vi "To Scaled Value.vi"(8 "error in":errorcluster, 10 "Response":string) -> (0 "error out":errorcluster, 1 "Unit":T1, 2 "Scaled Value":dbl format="%#.6f")   [LabVIEW 2018, in "Mercury iXX.lvlib"]
doc: "This VI converts the raw string value provided by the instrument into a scaled numeric (i.e. without prefix) and a unit string."
uses:
  Mercury iXX.lvlib
  Unit String.ctl
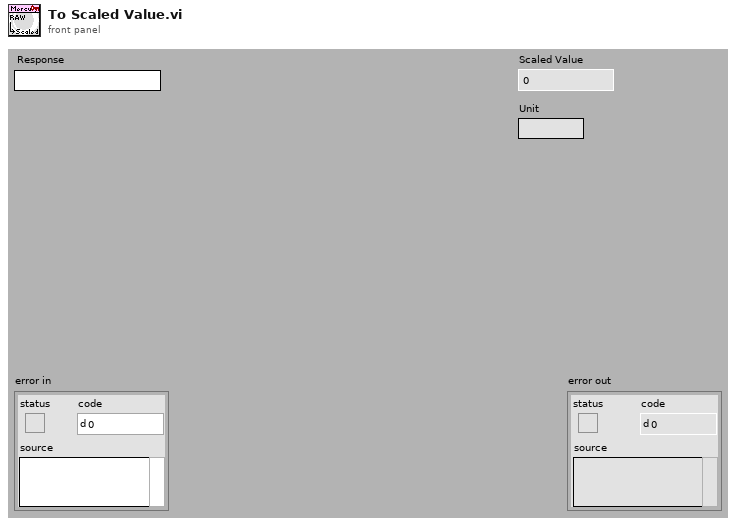
[diagram p1: front panel]
types:
  T1 = typedef "Mercury iXX.lvlib/Unit String.ctl" = string
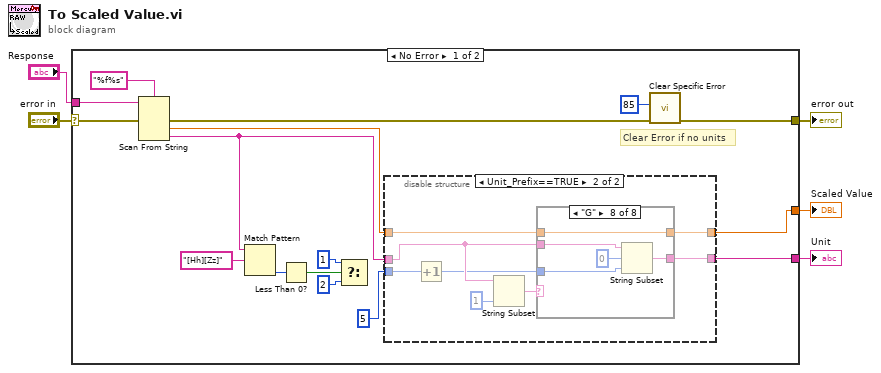
[diagram p0: block diagram]
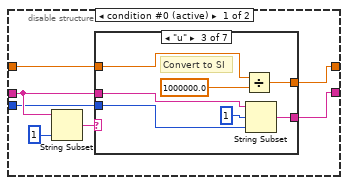
[diagram p2: hidden frame]
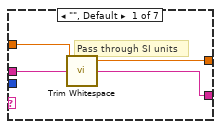
[diagram p3: hidden frame]
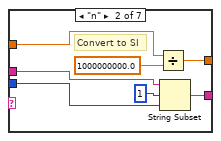
[diagram p4: hidden frame]
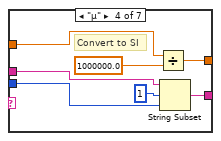
[diagram p5: hidden frame]
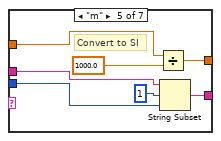
[diagram p6: hidden frame]
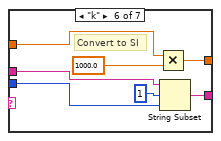
[diagram p7: hidden frame]
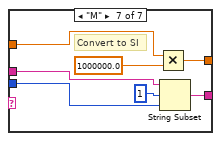
[diagram p8: hidden frame]
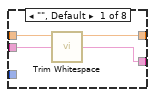
[diagram p9: hidden frame]
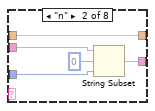
[diagram p10: hidden frame]
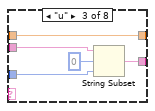
[diagram p11: hidden frame]
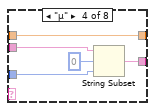
[diagram p12: hidden frame]
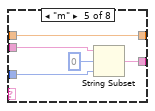
[diagram p13: hidden frame]
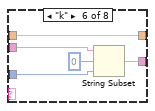
[diagram p14: hidden frame]
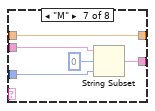
[diagram p15: hidden frame]
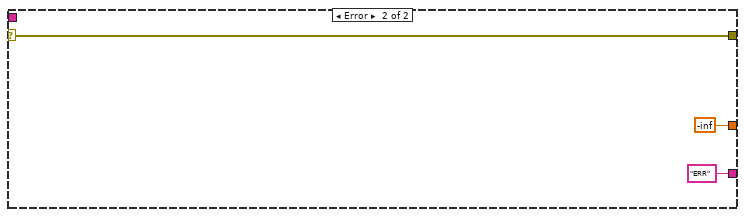
[diagram p16: hidden frame]
diagram:
  n1 = case shown="No Error" "error in" {
    selector: "error in" -> [w17 w122]
    tunnel: [w15 w122] -> w4
    tunnel: "Response" -> [w7 _]
    tunnel: [w19 -inf] -> w2
    tunnel: [w18 "ERR" ("Unit-")] -> w1
    frame No Error {
      # "Clear Error if no units"
      n2 = Scan From String(format string="%f%s", input string=w7, error in=w17) -> (error out=w16:errorcluster, output 1=w20:dbl, output 2=w13:string)  [unwired: 1 in, 4 out]
      n3 = Match Pattern(string=w13, regular expression="[Hh][Zz]") -> (offset past match=w11:i32)  [unwired: 4 out]
      n4 = Less Than 0?(x=w11) -> (x < 0?=w10:bool)
      n5 = Select(t=1 ("length (rest)"), s=w10, f=2) -> ()  [unwired: 1 out]
      n6 = disable-structure shown="Unit_Prefix==TRUE" {
        disable-tunnel: w20 -> [w26 w78]
        disable-tunnel: [w25 w77] -> w19
        disable-tunnel: [w24 w76] -> w18
        disable-tunnel: w13 -> [w23 w79]
        disable-tunnel: 5 ("length (rest)") -> [w22 w75]
        frame condition #0 (active) {
          n7 = String Subset(string=w23, length (rest)=1 ("length (rest)")) -> (substring=w27:string)  [unwired: 1 out]
          n8 = case shown="\"u\"" w27 {
            tunnel: w26 -> [w31 w38 w45 w52 w59 w66 w73]
            tunnel: [w31 w36 w43 w50 w57 w64 w71] -> w25
            tunnel: w23 -> [w30 w35 w42 w49 w56 w63 w70]
            tunnel: [w29 w33 w40 w47 w54 w61 w68] -> w24
            tunnel: w22 -> [_ w32 w39 w46 w53 w60 w67]
            frame "", Default {
              # "Pass through SI units"
              n9 = call "Trim Whitespace.vi"("string"=w30) -> ("trimmed string"=w29:string)  [unwired: 1 in]
            }
            frame "n" {
              # "Convert to SI"
              n10 = Divide(x=w38, y=1000000000.0) -> (x/y=w36:dbl)
              n11 = String Subset(string=w35, offset (0)=1 ("length (rest)"), length (rest)=w32) -> (substring=w33:string)
            }
            frame "u" {
              # "Convert to SI"
              n12 = Divide(x=w45, y=1000000.0) -> (x/y=w43:dbl)
              n13 = String Subset(string=w42, offset (0)=1 ("length (rest)"), length (rest)=w39) -> (substring=w40:string)
            }
            frame "µ" {
              # "Convert to SI"
              n14 = Divide(x=w52, y=1000000.0) -> (x/y=w50:dbl)
              n15 = String Subset(string=w49, offset (0)=1 ("length (rest)"), length (rest)=w46) -> (substring=w47:string)
            }
            frame "m" {
              # "Convert to SI"
              n16 = Divide(x=w59, y=1000.0) -> (x/y=w57:dbl)
              n17 = String Subset(string=w56, offset (0)=1 ("length (rest)"), length (rest)=w53) -> (substring=w54:string)
            }
            frame "k" {
              # "Convert to SI"
              n18 = Multiply(x=w66, y=1000.0) -> (x*y=w64:dbl)
              n19 = String Subset(string=w63, offset (0)=1 ("length (rest)"), length (rest)=w60) -> (substring=w61:string)
            }
            frame "M" {
              # "Convert to SI"
              n20 = Multiply(x=w73, y=1000000.0) -> (x*y=w71:dbl)
              n21 = String Subset(string=w70, offset (0)=1 ("length (rest)"), length (rest)=w67) -> (substring=w68:string)
            }
          }
        }
        frame condition #1 {
          n22 = Increment(x=w75) -> (x+1=w74:i32)
          n23 = String Subset(string=w79, length (rest)=1 ("length (rest)")) -> (substring=w80:string)  [unwired: 1 out]
          n24 = case shown="\"G\"" w80 {
            tunnel: w78 -> [w84 w86 w90 w95 w100 w105 w110 w119]
            tunnel: [w84 w86 w90 w95 w100 w105 w110 w119] -> w77
            tunnel: w79 -> [w83 w89 w94 w99 w104 w109 w114 w117]
            tunnel: [w82 w87 w92 w97 w102 w107 w112 w115] -> w76
            tunnel: w74 -> [_ w85 w91 w96 w101 w106 w111 w116]
            frame "", Default {
              n25 = call "Trim Whitespace.vi"("string"=w83) -> ("trimmed string"=w82:string)  [unwired: 1 in]
            }
            frame "n" {
              n26 = String Subset(string=w89, offset (0)=0 ("length (rest)"), length (rest)=w85) -> (substring=w87:string)
            }
            frame "u" {
              n27 = String Subset(string=w94, offset (0)=0 ("length (rest)"), length (rest)=w91) -> (substring=w92:string)
            }
            frame "µ" {
              n28 = String Subset(string=w99, offset (0)=0 ("length (rest)"), length (rest)=w96) -> (substring=w97:string)
            }
            frame "m" {
              n29 = String Subset(string=w104, offset (0)=0 ("length (rest)"), length (rest)=w101) -> (substring=w102:string)
            }
            frame "k" {
              n30 = String Subset(string=w109, offset (0)=0 ("length (rest)"), length (rest)=w106) -> (substring=w107:string)
            }
            frame "M" {
              n31 = String Subset(string=w114, offset (0)=0 ("length (rest)"), length (rest)=w111) -> (substring=w112:string)
            }
            frame "G" {
              n32 = String Subset(string=w117, offset (0)=0 ("length (rest)"), length (rest)=w116) -> (substring=w115:string)
            }
          }
        }
      }
      n33 = call "Clear Specific Error.vi"("error in"=w16, "Code (-1:All)"=85) -> ("error out"=w15:errorcluster)  [unwired: 9 out]
    }
    frame Error {
    }
  }
  "error out" <- w4
  "Scaled Value" <- w2
  "Unit" <- w1
